vi "automatic_step_submit.vi"(7 "transition_queue":refnum<queue>, 8 "error in (no error)":errorcluster, 10 "data":variant, 11 "recipe_data":variant) -> (0 "error out":errorcluster)   [LabVIEW 2015, in "lv-recipe-machine.lvlib" / "example_02.lvlib"]
uses:
  example_02.lvlib
  public/_controls/transition.ctl
  _controls/customer.ctl
  lv-recipe-machine.lvlib
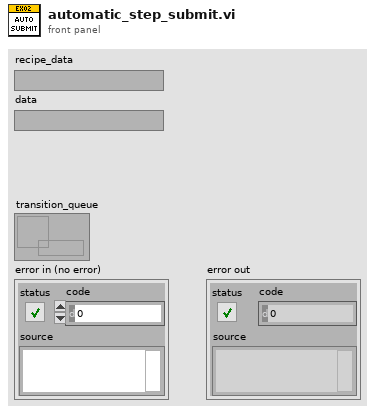
[diagram p1: front panel]
types:
  T1 = typedef "lv-recipe-machine.lvlib/example_02.lvlib/customer.ctl" = cluster{"first_name":string, "last_name":string, "address_1":string, "address_2":string, "city":string, "state":string, "zip_code":string}
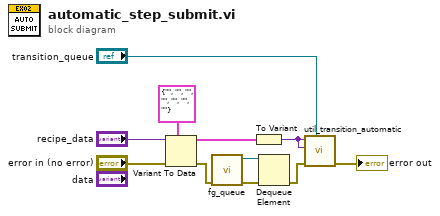
[diagram p0: block diagram]
diagram:
  n1 = Variant To Data(error in="error in (no error)", type=T1 {"first_name"="", "last_name"="", "address_1"="", "address_2"="", "city"="", "state"="", "zip_code"=""} ("customer"), Variant="recipe_data") -> (data=w3:T1, error out=w6:errorcluster)
  n2 = call "fg_queue.vi"("error in (no error)"=w6) -> ("error out"=w4:errorcluster, "queue out"=w5:refnum<queue>)  [unwired: 9 in]
  n3 = To Variant(anything=w3) -> (Variant=w1:variant)
  n4 = Dequeue Element(queue=w5, error in (no error)=w4) -> (error out=w2:errorcluster)  [unwired: 1 in, 3 out]
  n5 = call "util_transition_automatic.vi"("transition_queue"="transition_queue", "error in (no error)"=w2, "data"=w1, "recipe_data"=w1) -> ("error out"=→"error out":errorcluster)  [unwired: 7 in]
